vi "BT DUT RX Configure.vi"(0 "niDTS BT DUT in":refnum<class "niDTS BT Dut.lvclass">, 11 "error in (no error)":errorcluster) -> (4 "niDTS BT DUT out":refnum<class "niDTS BT Dut.lvclass">, 15 "error out":errorcluster)   [LabVIEW 2015, in "niDTS BT.lvlib" / "niDTS BT Dut.lvclass"]
uses:
  niDTS BT Dut.lvclass
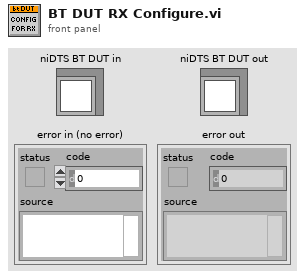
[diagram p1: front panel]
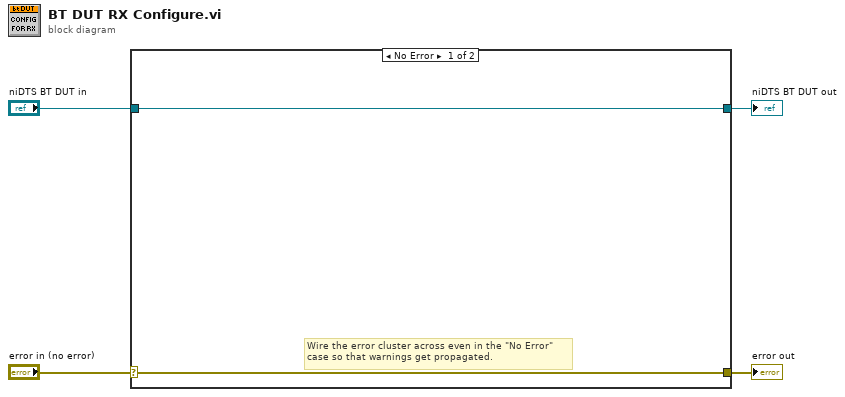
[diagram p0: block diagram]
diagram:
  n1 = case shown="No Error" "error in (no error)" {
    selector: "error in (no error)" -> [w5 w8]
    tunnel: [w5 w8] -> w3
    tunnel: [w6 w7] -> w1
    tunnel: "niDTS BT DUT in" -> [w6 w7]
    frame No Error {
      # "Wire the error cluster across even in the \"No Error\"\ncase so that warnings get propagated."
    }
    frame Error {
    }
  }
  "error out" <- w3
  "niDTS BT DUT out" <- w1
